vi "Set value by Variant.vi"(8 "error in (no error)":errorcluster, 10 "Variant":variant, 11 "Column in":refnum<class "Text Field.lvclass">) -> (0 "error out":errorcluster, 3 "Column out":refnum<class "Text Field.lvclass">)   [LabVIEW 2020]
uses:
  Text Field.lvclass
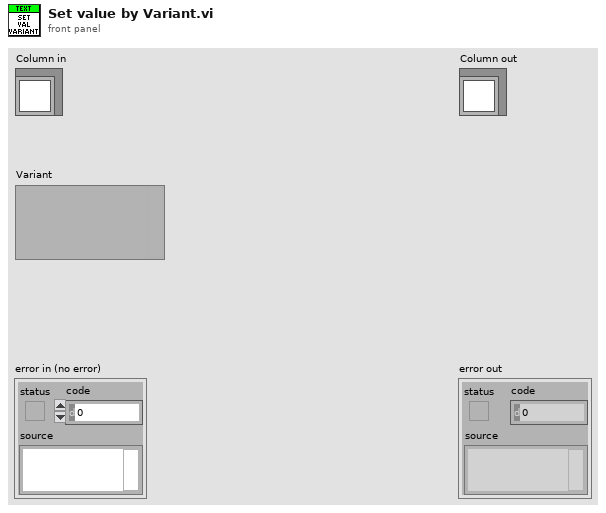
[diagram p1: front panel]
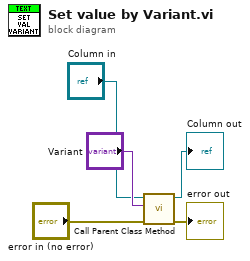
[diagram p0: block diagram]
diagram:
  n1 = call-parent "Call Parent Class Method"("error in (no error)"="error in (no error)", "Variant"="Variant", "Column in"="Column in") -> ("error out"=→"error out":errorcluster, "Column out"=→"Column out":refnum<class "Text Field.lvclass">)  [unwired: 7 in]
